vi "TC560-Command Data(FGV).vi"(6 "File Method":T3, 8 "error in":errorcluster, 11 "Configuration In":T1={"Connection Setting"={"VISA Resource Name"="", "Baud Rate"=9600, "Parity"=0, "Flow Control"=0}, "Wait For Read"=0} {"Connection Setting"."Flow Control" items=["None", "XON/XOFF", "RTS/CTS", "XON/XOFF & RTS/CTS", "DTR/DSR", "XON/XOFF & DTR/DSR"]; "Connection Setting"."Parity" items=["None", "Odd", "Even", "Mark", "Space"]; "Connection Setting"."Baud Rate" items=["2400"=2400, "4800"=4800, "9600"=9600]}) -> (0 "error out":errorcluster, 3 "Configuration Out":T1={"Connection Setting"={"VISA Resource Name"="", "Baud Rate"=9600, "Parity"=0, "Flow Control"=0}, "Wait For Read"=0} {"Connection Setting"."Flow Control" items=["None", "XON/XOFF", "RTS/CTS", "XON/XOFF & RTS/CTS", "DTR/DSR", "XON/XOFF & DTR/DSR"]; "Connection Setting"."Parity" items=["None", "Odd", "Even", "Mark", "Space"]; "Connection Setting"."Baud Rate" items=["2400"=2400, "4800"=4800, "9600"=9600]})   [LabVIEW 2018]
uses:
  Data Def/TC560-File Method.ctl
  Data Def/TC560-Configuration.ctl
  Data Def/TC560-Connection Setting.ctl
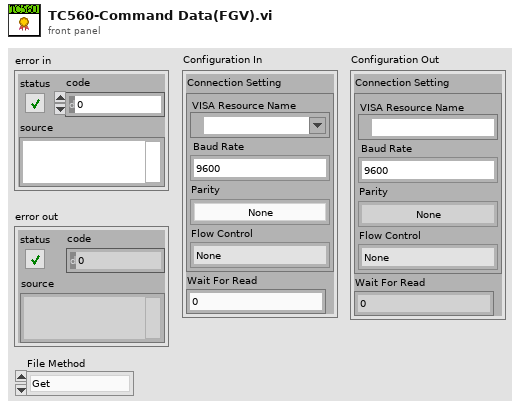
[diagram p1: front panel]
types:
  T1 = typedef "TC560-Configuration.ctl" = cluster{"Connection Setting":T2, "Wait For Read":u32}
  T2 = typedef "TC560-Connection Setting.ctl" = cluster{"VISA Resource Name":refnum<visa-resource-name>, "Baud Rate":u32, "Parity":u16, "Flow Control":u16}
  T3 = typedef "TC560-File Method.ctl" = enum16{"Get", "Put", "Load", "Save"}
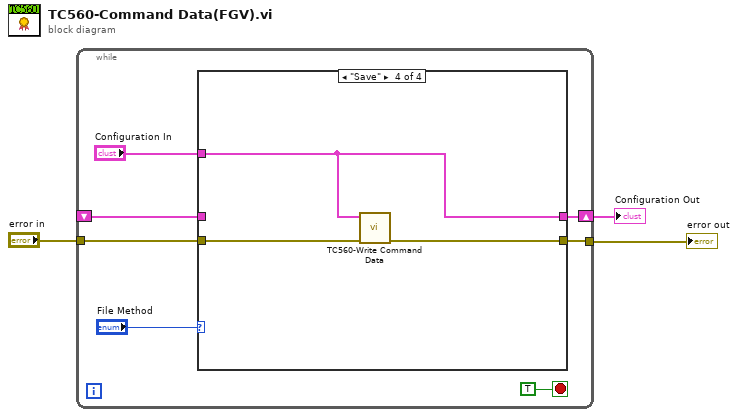
[diagram p0: block diagram]
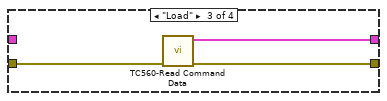
[diagram p4: hidden frame]
diagram:
  n1 = while {
    tunnel: [w8] -> w1
    shift-right: [w7] -> w2
    shift-left: _ -> [w6]
    tunnel: "error in" -> [w5]
    stop <- TRUE stop-if-true
    n2 = case shown="\"Save\"" "File Method" {
      tunnel: [w11 w13 w17 w19] -> w8
      tunnel: [w12 w14 w16 w18] -> w7
      tunnel: w6 -> [w12 _ _ _]
      tunnel: w5 -> [w11 w13 w15 w20]
      tunnel: "Configuration In" -> [_ w14 _ w18]
      frame "Get", Default {
      }
      frame "Put" {
      }
      frame "Load" {
        n3 = call "TC560-Read Command Data.vi"("error in"=w15) -> ("error out"=w17:errorcluster, "Configuration"=w16:T1)  [unwired: 9 in]
      }
      frame "Save" {
        n4 = call "TC560-Write Command Data.vi"("error in"=w20, "Configuration"=w18) -> ("error out"=w19:errorcluster)  [unwired: 9 in]
      }
    }
  }
  "error out" <- w1
  "Configuration Out" <- w2
